vi "adc_read1.vi"() -> ()   [LabVIEW 2018]
uses:
  <vilib>/Instr/_visa.llb/VISA Configure Serial Port (Instr).vi
  <vilib>/Utility/file.llb/Write Delimited Spreadsheet (DBL).vi
panel:
  out "数值":i32
  out "数组 3":dbl[](array[numeric])
  out "数组":dbl[](array[numeric])
  out "VISA resource name out":refnum<visa-resource-name>
  out "数组 2":dbl[](array[numeric])
  in  "second":dbl=600.0
  in  "first":dbl=400.0
  in  "offset":dbl=80.0
  in  "mode":dbl
  in  "fpga":refnum<visa-resource-name>="COM14" caption="VISA资源名称"
  in  "平均次数":dbl=1.0
  in  "low_time":dbl=40.0
  in  "high_time":dbl=40.0
  in  "start_time":dbl
  in  "频率":dbl=2870.0
  out "时域":cluster{dbl[], dbl[]}(graph)={[0.0, 8.0, 16.0, 24.0, 32.0, 40.0, 48.0, 56.0, 64.0, 72.0], [0.035591, 0.035591, 0.035591, 0.035591, 0.035591, 0.035591, 0.035591, 0.035591, 0.035591, 0.035591]}
  out "时域读取 3":string="ADF_Set_Freq 2870\r\n\r\nQuantax:/$ Pulse_Ctrl 0 40 40 0 80 400 600\r\n\r\nQuantax:/$ ADC_Start 1\r\n+0.039597\r\r\n+0.035591\r\r\n+0.030479\r\r\n+0.027428\r\r\n+0.027504\r\r\n+0.029449\r\r\n+0.034523\r\r\n+0.039253\r\r\n+0.041847\r\r\n+0.040741\r\r\n"
  out "返回数 3":u32=211
  out "x+y 3":dbl=211.0
  out "时域截取 3":string="+0.039597\r\r\n+0.035591\r\r\n+0.030479\r\r\n+0.027428\r\r\n+0.027504\r\r\n+0.029449\r\r\n+0.034523\r\r\n+0.039253\r\r\n+0.041847\r\r\n+0.040741\r\r\n"
  out "连接的字符串 3":string="ADC_Start 1\r"
  out "点数 2":dbl=10.0
  out "请求读取字节数 2":dbl=6080.0
  out "连接的字符串 5":string="Pulse_Ctrl 0 40 40 0 80 400 600\r"
  out "长度 2":i32=32
  out "连接的字符串 4":string="ADF_Set_Freq 2870\r"
  out "长度":i32=18
  in  "时域荧光":path=path "D:/Test.txt"
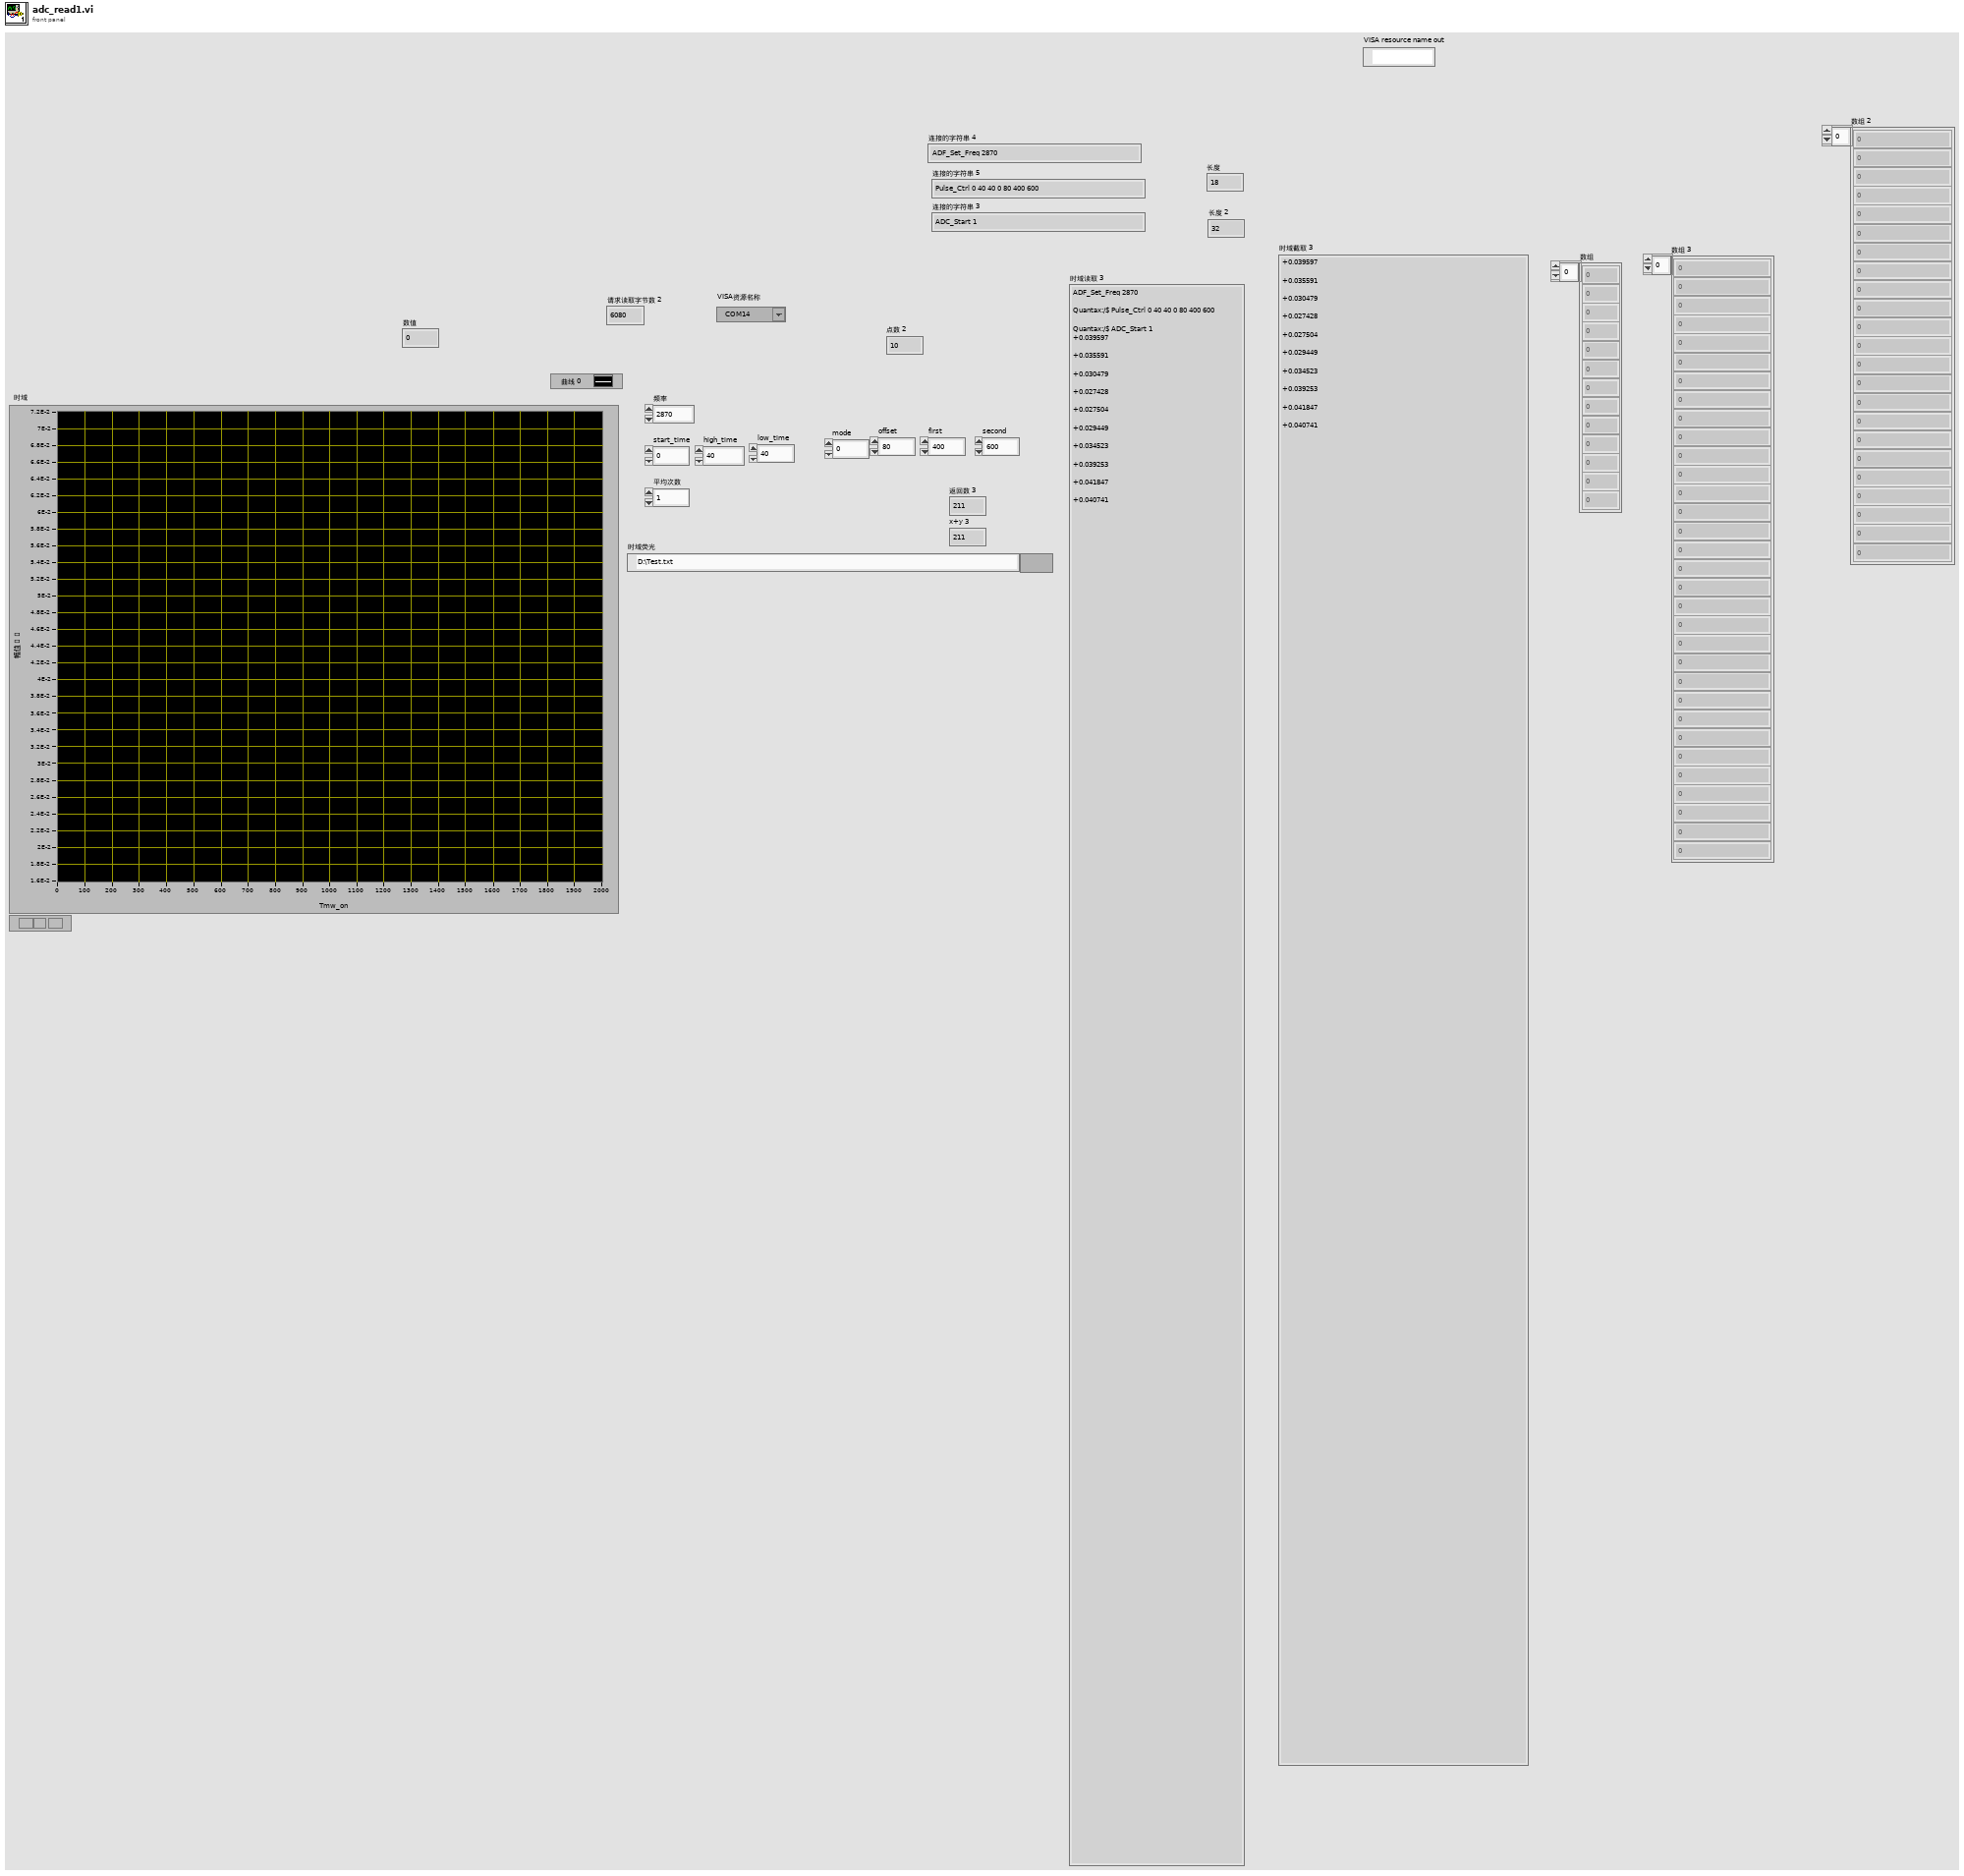
[diagram p1: front panel]
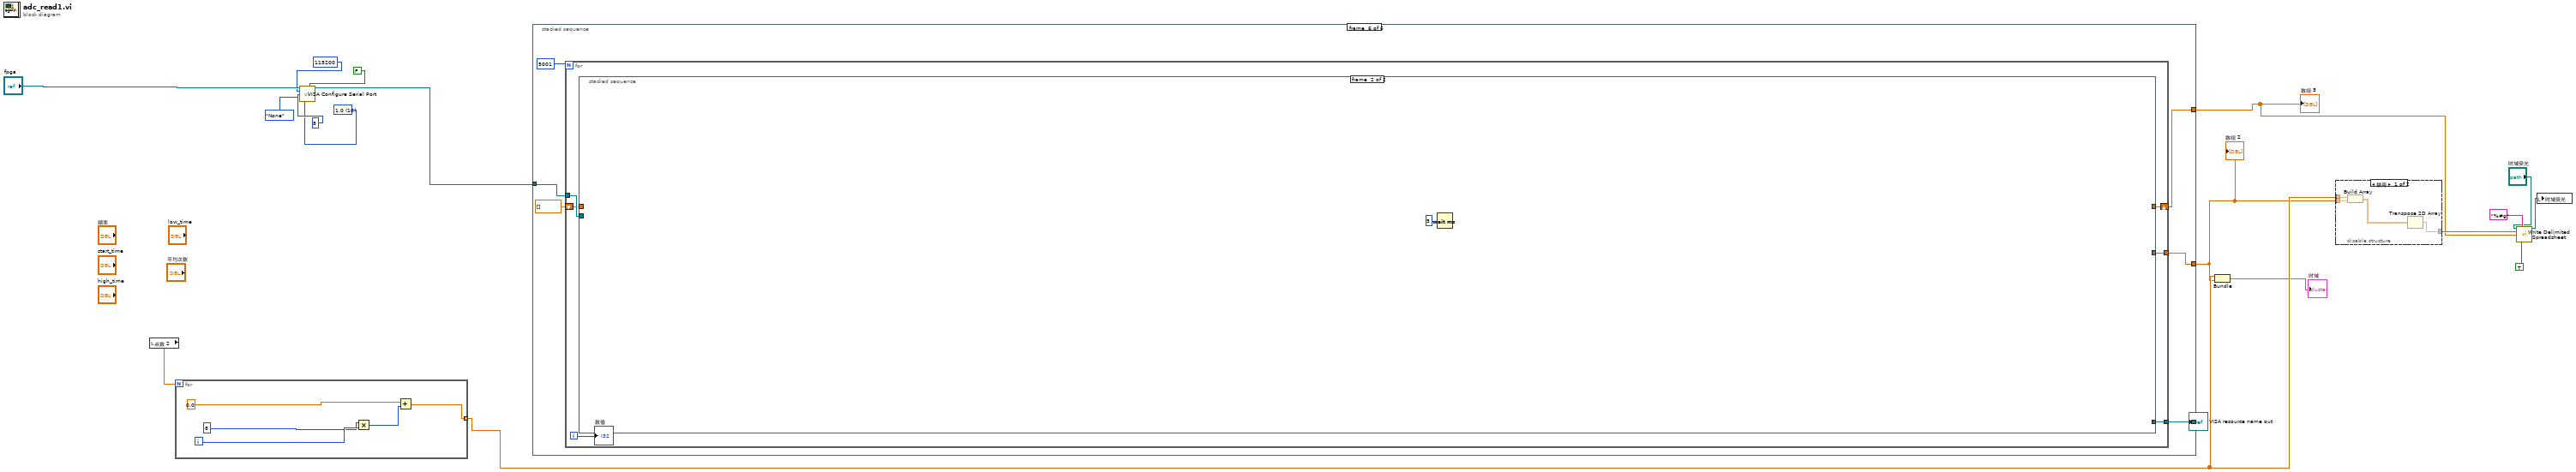
[diagram p0: block diagram]
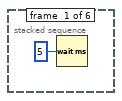
[diagram p3: hidden frame]
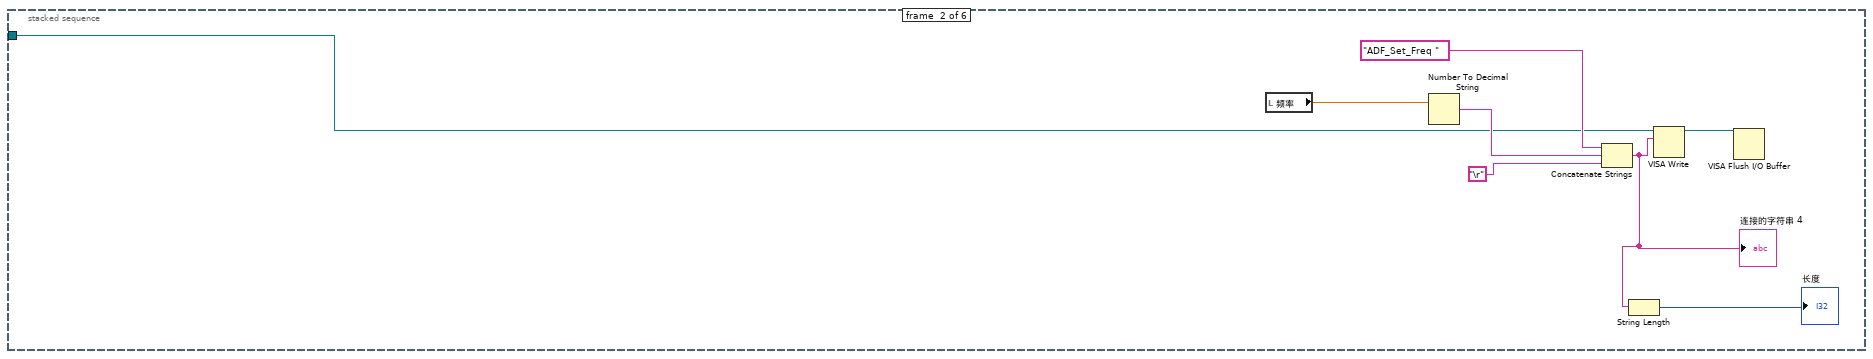
[diagram p4: hidden frame]
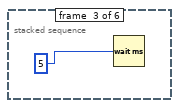
[diagram p5: hidden frame]
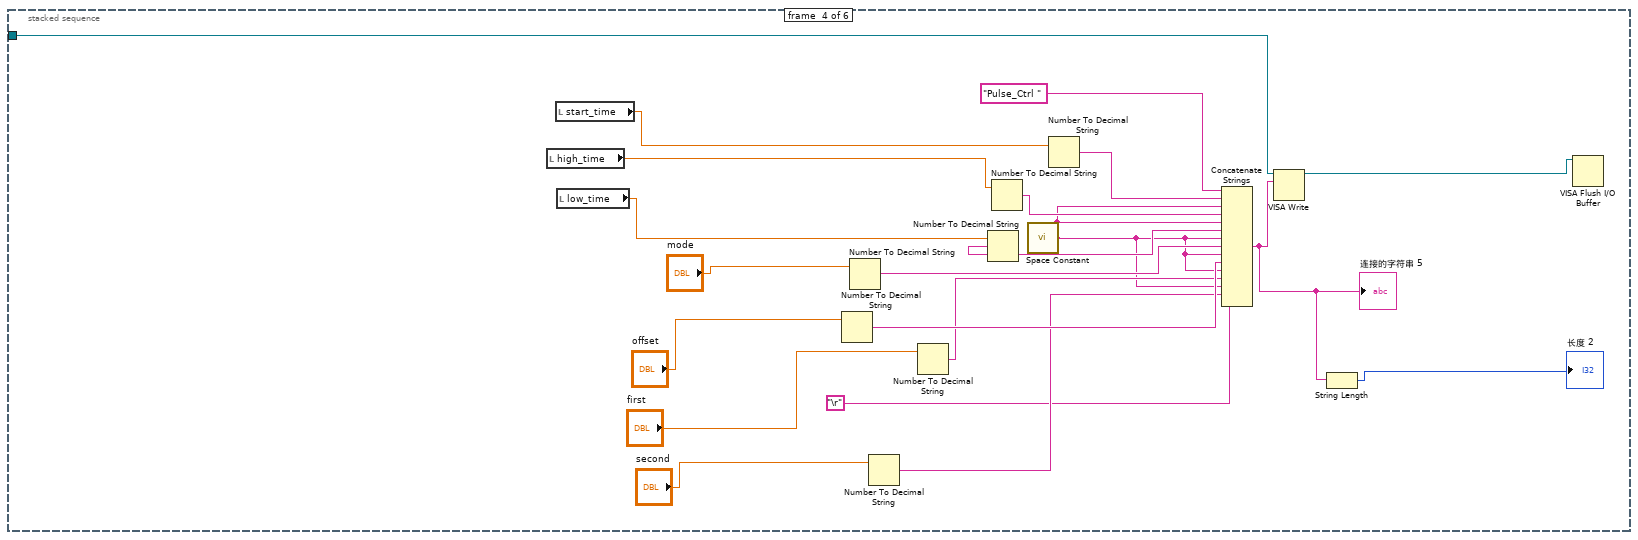
[diagram p6: hidden frame]
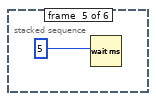
[diagram p7: hidden frame]
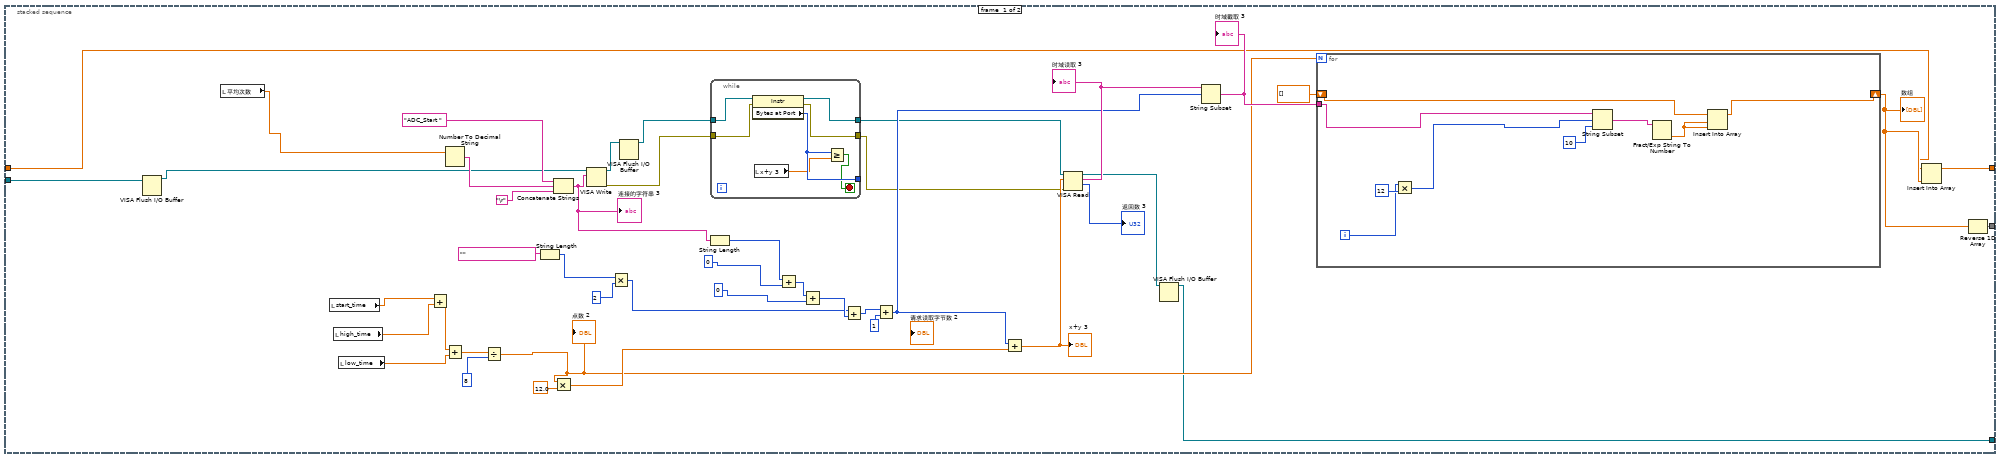
[diagram p8: hidden frame]
diagram:
  w13 = u16 10 items=["1.0"=10, "1.5"=15, "2.0"=20] ("stop bits (10: 1 bit)")
  n1 = local read "点数 2"() -> (w8:dbl)
  n2 = for {
    N: w8 -> [_]
    tunnel: [w21] -> w7 mode=indexing
    i -> [w23]
    n3 = Multiply(x=8, y=w23) -> (x*y=w22:i32)
    n4 = Add(x=0.0, y=w22) -> (x+y=w21:dbl)
  }
  n5 = call-poly "VISA Configure Serial Port"("VISA resource name"="fpga", "Enable Termination\nChar (T)"=FALSE, "baud rate (9600)"=u32 115200, "data bits (8)"=u16 8, "parity (0:none)"=enum16{"None", "Odd", "Even", "Mark", "Space"}."None", "stop bits (10: 1 bit)"=w13) -> ("VISA resource name out"=w9:refnum<visa-resource-name>)  [unwired: 8 in, 1 out]
  n6 = stacked-sequence {
    tunnel: w9 -> [_ w30 _ w47 _ w61]
    tunnel: [_ _ _ _ _ w60] -> w4
    tunnel: [_ _ _ _ _ w58] -> w2
    tunnel: [_ _ _ _ _ w56] -> w1
    frame #0 {
      n7 = Wait (ms)(milliseconds to wait=u32 5 ("等待时间（毫秒）")) -> ()  [unwired: 1 out]
    }
    frame #1 {
      n8 = local read "频率"() -> (w29:dbl)
      n9 = Number To Decimal String(number=w29) -> (decimal integer string=w31:string)  [unwired: 1 in]
      n10 = Concatenate Strings("ADF_Set_Freq ", w31, "\r") -> (w27:string)
      "连接的字符串 4" <- w27
      n11 = String Length(string=w27) -> (length=→"长度":i32)
      n12 = VISA Write(VISA resource name=w30, write buffer=w27) -> (VISA resource name out=w25:refnum<visa-resource-name>)  [unwired: 1 in, 2 out]
      n13 = VISA Flush I/O Buffer(VISA resource name=w25) -> ()  [unwired: 2 in, 2 out]
    }
    frame #2 {
      n14 = Wait (ms)(milliseconds to wait=5) -> ()  [unwired: 1 out]
    }
    frame #3 {
      n15 = local read "high_time"() -> (w51:dbl)
      n16 = local read "start_time"() -> (w52:dbl)
      n17 = local read "low_time"() -> (w49:dbl)
      n18 = Number To Decimal String(number="offset") -> (decimal integer string=w39:string)  [unwired: 1 in]
      n19 = Number To Decimal String(number="mode") -> (decimal integer string=w43:string)  [unwired: 1 in]
      n20 = Number To Decimal String(number="second") -> (decimal integer string=w36:string)  [unwired: 1 in]
      n21 = Number To Decimal String(number="first") -> (decimal integer string=w38:string)  [unwired: 1 in]
      n22 = Number To Decimal String(number=w49) -> (decimal integer string=w48:string)  [unwired: 1 in]
      n23 = Number To Decimal String(number=w51) -> (decimal integer string=w50:string)  [unwired: 1 in]
      n24 = call <vilib>:"Space Constant.vi"() -> ("String"=w37:string)
      n25 = Number To Decimal String(number=w52) -> (decimal integer string=w53:string)  [unwired: 1 in]
      n26 = Concatenate Strings("Pulse_Ctrl ", w53, w37, w50, w37, w48, w37, w43, w37, w39, w37, w38, w37, w36, "\r") -> (w46:string)
      "连接的字符串 5" <- w46
      n27 = VISA Write(VISA resource name=w47, write buffer=w46) -> (VISA resource name out=w34:refnum<visa-resource-name>)  [unwired: 1 in, 2 out]
      n28 = String Length(string=w46) -> (length=→"长度 2":i32)
      n29 = VISA Flush I/O Buffer(VISA resource name=w34) -> ()  [unwired: 2 in, 2 out]
    }
    frame #4 {
      n30 = Wait (ms)(milliseconds to wait=5) -> ()  [unwired: 1 out]
    }
    frame #5 {
      n31 = for {
        N: 5001 -> [_]
        tunnel: [w67] -> w60
        tunnel: w61 -> [w66]
        tunnel: [w65] -> w58
        shift-right: [w64] -> w56
        shift-left: dbl[] [] -> [w63]
        i -> [w62]
        n32 = stacked-sequence {
          tunnel: [w79 _] -> w67
          tunnel: w66 -> [w74 _]
          tunnel: [w77 _] -> w65
          tunnel: [w70 _] -> w64
          tunnel: w63 -> [w68 _]
          frame #0 {
            n33 = VISA Flush I/O Buffer(VISA resource name=w74) -> (VISA resource name out=w73:refnum<visa-resource-name>)  [unwired: 2 in, 1 out]
            n34 = local read "平均次数"() -> (w95:dbl)
            n35 = local read "start_time"() -> (w101:dbl)
            n36 = local read "high_time"() -> (w100:dbl)
            n37 = local read "low_time"() -> (w99:dbl)
            n38 = Add(x=w101, y=w100) -> (x+y=w98:dbl)
            n39 = Number To Decimal String(number=w95) -> (decimal integer string=w103:string)  [unwired: 1 in]
            n40 = Add(x=w98, y=w99) -> (x+y=w97:dbl)
            n41 = Divide(x=w97, y=8) -> (x/y=w86:dbl)
            "点数 2" <- w86
            n42 = String Length(string="") -> (length=w89:i32)
            n43 = Concatenate Strings("ADC_Start ", w103, "\r") -> (w94:string)
            "连接的字符串 3" <- w94
            n44 = Multiply(x=w86, y=12.0) -> (x*y=w106:dbl)
            n45 = VISA Write(VISA resource name=w73, write buffer=w94) -> (VISA resource name out=w72:refnum<visa-resource-name>, error out=w82:errorcluster)  [unwired: 1 in, 1 out]
            n46 = Multiply(x=w89, y=2) -> (x*y=w87:i32)
            n47 = VISA Flush I/O Buffer(VISA resource name=w72) -> (VISA resource name out=w71:refnum<visa-resource-name>)  [unwired: 2 in, 1 out]
            n48 = String Length(string=w94) -> (length=w93:i32)
            n49 = while {
              tunnel: [w114] -> _
              tunnel: w71 -> [w118]
              tunnel: [w117] -> w81
              tunnel: w82 -> [w116]
              tunnel: [w115] -> w80
              stop <- w112 stop-if-true
              n50 = property class="Instr"(reference=w118, error in=w116) -> (reference out=w117:refnum<visa-resource-name>, error out=w115:errorcluster, "Bytes at Port"=w114:u32)
              n51 = local read "x+y 3"() -> (w113:dbl)
              n52 = Greater Or Equal?(x=w114, y=w113) -> (x >= y?=w112:bool)
            }
            n53 = Add(x=w93, y=0) -> (x+y=w92:i32)
            n54 = Add(x=w92, y=0) -> (x+y=w90:i32)
            n55 = Add(x=w87, y=w90) -> (x+y=w85:i32)
            n56 = Add(x=w85, y=1) -> (x+y=w83:i32)
            n57 = Add(x=w83, y=w106) -> (x+y=w104:dbl)
            "x+y 3" <- w104
            n58 = VISA Read(VISA resource name=w81, byte count=w104, error in (no error)=w80) -> (VISA resource name out=w78:refnum<visa-resource-name>, read buffer=w109:string, return count=→"返回数 3":u32)  [unwired: 1 out]
            "时域读取 3" <- w109
            n59 = VISA Flush I/O Buffer(VISA resource name=w78) -> (VISA resource name out=w77:refnum<visa-resource-name>)  [unwired: 2 in, 1 out]
            n60 = String Subset(string=w109, offset (0)=w83) -> (substring=w108:string)  [unwired: 1 in]
            "时域截取 3" <- w108
            n61 = for {
              N: w86 -> [_]
              tunnel: w108 -> [w122]
              shift-right: [w127] -> w69
              shift-left: dbl[] [] -> [w126]
              i -> [w120]
              n62 = Multiply(x=w120, y=12) -> (x*y=w119:i32)
              n63 = String Subset(string=w122, offset (0)=w119, length (rest)=10 ("长度（剩余）")) -> (substring=w125:string)
              n64 = Fract/Exp String To Number(string=w125) -> (number=w121:dbl)  [unwired: 3 in, 1 out]
              n65 = Insert Into Array(array=w126, index=w121, new element=w121) -> (w127:dbl[])
            }
            "数组" <- w69
            n66 = Insert Into Array(array=w68, new element=w69) -> (w70:dbl[])  [unwired: 1 in]
            n67 = Reverse 1D Array(array=w69) -> (reversed array=w79:dbl[])
          }
          frame #1 {
            n68 = Wait (ms)(milliseconds to wait=u32 5 ("等待时间（毫秒）")) -> ()  [unwired: 1 out]
          }
        }
        "数值" <- w62
      }
    }
  }
  "数组 2" <- w4
  "VISA resource name out" <- w2
  "数组 3" <- w1
  n69 = Bundle(w7, w4) -> (→"时域":cluster{dbl[], dbl[]})  [unwired: 1 in]
  n70 = disable-structure shown="禁用" {
    disable-tunnel: w7 -> [w132 _]
    disable-tunnel: w4 -> [w131 _]
    disable-tunnel: [w129 _] -> w6
    frame Disabled {
      n71 = Build Array(w132, w131) -> (w130:dbl[][])
      n72 = Transpose 2D Array(2D array=w130) -> (transposed array=w129:dbl[][])
    }
    frame Enabled {
    }
  }
  n73 = call-poly <vilib>:"Write Delimited Spreadsheet.vi"("file path (dialog if empty)"="时域荧光", "format (%.3f)"="%#g", "2D data"=w6, "1D data"=w1, "transpose? (no:F)"=TRUE) -> ("new file path (Not A Path if cancelled)"=w10:path)  [unwired: 9 in, 1 out]
  n74 = local write "时域荧光"(w10) -> ()
